vi "File Save.vi"(0 "Cancel Button":bool, 1 "Save Button":bool, 8 "error in":errorcluster, 11 "Path":path) -> (2 "error out":errorcluster, 3 "refnum out":refnum<file>, 4 "File Name 2":string, 6 "Cancelled":bool=TRUE)   [LabVIEW 2020]
panel:
  in  "File Name":string
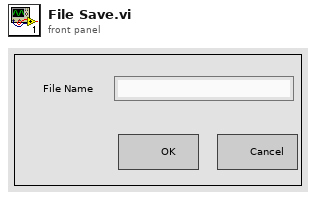
[diagram p1: front panel]
types:
  T1 = enum16{"open", "replace", "create", "open or create", "replace or create", "replace or create with confirmation"}
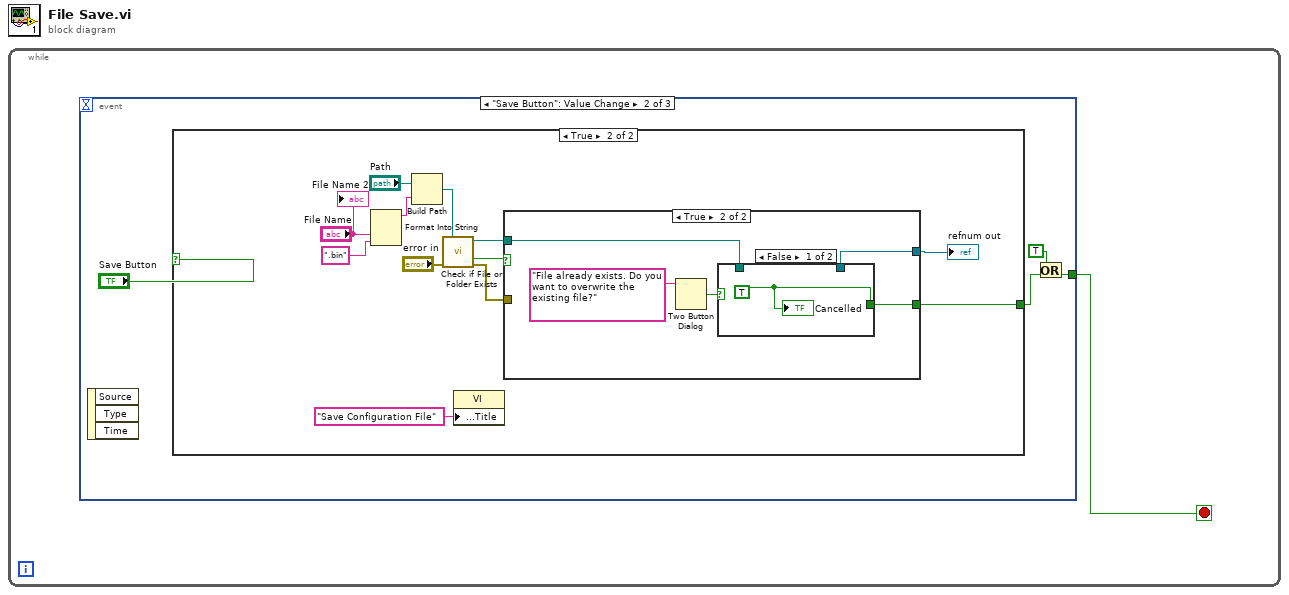
[diagram p0: block diagram]
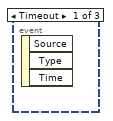
[diagram p2: hidden frame]
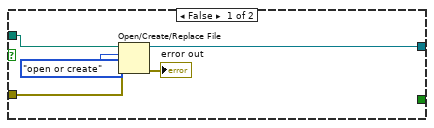
[diagram p4: hidden frame]
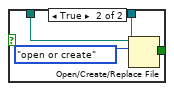
[diagram p5: hidden frame]
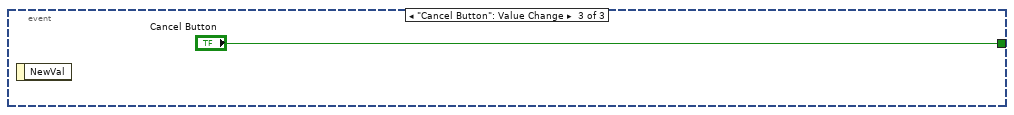
[diagram p6: hidden frame]
diagram:
  n1 = while {
    stop <- w1 stop-if-true
    n2 = event shown="[1] \"Save Button\": Value Change" {
      selector: _ -> [_ _ _]
      dyn-events: _ -> [_ _ _]
      timeout: _ -> [_ _ _]
      tunnel: [_ w3 "Cancel Button"] -> w1
      event Timeout {
        n3 = event-data() -> ()  [unwired: 1 in, 3 out]
      }
      event "Save Button": Value Change {
        n4 = event-data() -> ()  [unwired: 1 in, 3 out]
        n5 = case shown="True" "Save Button" {
          tunnel: [_ w6] -> w4
          frame False {
          }
          frame True {
            n6 = Format Into String("File Name", ".bin" ("pattern (all files)")) -> (resulting string=w15:string)  [unwired: 3 in, 1 out]
            n7 = Build Path(base path="Path", name or relative path=w15) -> (appended path=w14:path)
            n8 = call <vilib>:"Check if File or Folder Exists.vi"("error in (no error)"="error in", "path"=w14) -> ("error out"=w12:errorcluster, "file or folder exists?"=w11:bool, "dup path"=w10:path)  [unwired: 7 in]
            n9 = property class="VI"("Front Panel.Title"="Save Configuration File" ("Front Panel Window:Title")) -> ()  [unwired: 2 in, 2 out]
            n10 = case shown="True" w11 {
              tunnel: w12 -> [w22 _]
              tunnel: w10 -> [w19 w25]
              tunnel: [w18 w24] -> w8
              tunnel: [_ w23] -> w6
              frame False {
                n11 = Open/Create/Replace File(file path (use dialog)=w19, error in=w22, operation (0:open)=T1."open or create") -> (refnum out=w18:refnum<file>, error out=→"error out":errorcluster)  [unwired: 3 in, 1 out]
              }
              frame True {
                n12 = Two Button Dialog(message="File already exists. Do you want to overwrite the existing file?") -> (T button?=w26:bool)  [unwired: 2 in]
                n13 = case shown="False" w26 {
                  tunnel: w25 -> [_ w31]
                  tunnel: [_ w30] -> w24
                  tunnel: [w28 _] -> w23
                  frame False {
                    w28 = TRUE
                    "Cancelled" <- w28
                  }
                  frame True {
                    n14 = Open/Create/Replace File(file path (use dialog)=w31, operation (0:open)=T1."open or create") -> (refnum out=w30:refnum<file>)  [unwired: 4 in, 2 out]
                  }
                }
              }
            }
            "refnum out" <- w8
            "File Name 2" <- "File Name"
          }
        }
        n15 = Or(x=TRUE, y=w4) -> (x .or. y?=w3:bool)
      }
      event "Cancel Button": Value Change {
        n16 = event-data() -> ()  [unwired: 1 in, 1 out]
      }
    }
  }
